vi "Application_SearchForComport.vi"(8 "error in":errorcluster, 11 "ComportNr":i32) -> (0 "error out":errorcluster, 3 "Found?":bool)   [LabVIEW 2016]
doc: "Searches the Windows Registry for a specific ComPort.\n\nAndreas Elmiger, 05.01.2017"
uses:
  <vilib>/Platform/system.llb/System Exec.vi
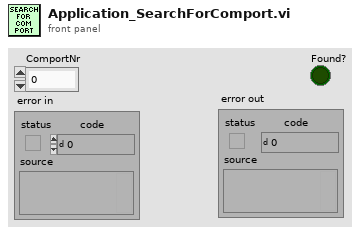
[diagram p1: front panel]
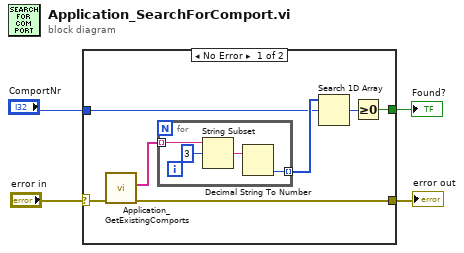
[diagram p0: block diagram]
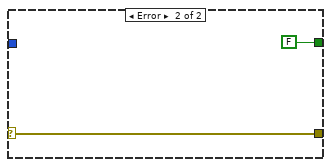
[diagram p2: hidden frame]
diagram:
  n1 = case shown="No Error" "error in" {
    selector: "error in" -> [w5 w16]
    tunnel: "ComportNr" -> [w9 _]
    tunnel: [w7 FALSE] -> w3
    tunnel: [w6 w16] -> w2
    frame No Error {
      n2 = call "Application_GetExistingComports.vi"("error in (no error)"=w5) -> ("error out"=w6:errorcluster, "Comport"=w11:string[])  [unwired: 8 in, 1 out]
      n3 = for {
        tunnel: w11 -> [w15] mode=indexing
        tunnel: [w12] -> w10 mode=indexing
        n4 = String Subset(string=w15, offset (0)=3) -> (substring=w13:string)  [unwired: 1 in]
        n5 = Decimal String To Number(string=w13) -> (number=w12:i32)  [unwired: 2 in, 1 out]
      }
      n6 = Search 1D Array(1D array=w10, element=w9) -> (index of element=w8:i32)  [unwired: 1 in]
      n7 = Greater Or Equal To 0?(x=w8) -> (x >= 0?=w7:bool)
    }
    frame Error {
    }
  }
  "Found?" <- w3
  "error out" <- w2
